vi "GetTriggerTime.vi"() -> (0 "error out":errorcluster, 3 "TriggerTime [ns]":i64)   [LabVIEW 2014]
uses:
  <vilib>/httpClient/LabVIEWHTTPClient.lvlib
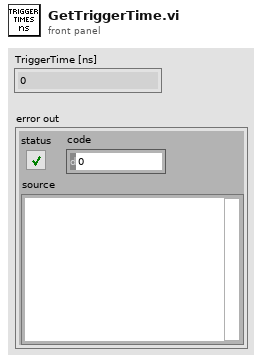
[diagram p1: front panel]
types:
  T1 = typedef "LabVIEWHTTPClient.lvlib/ClientHandle.ctl" = refnum<k1>
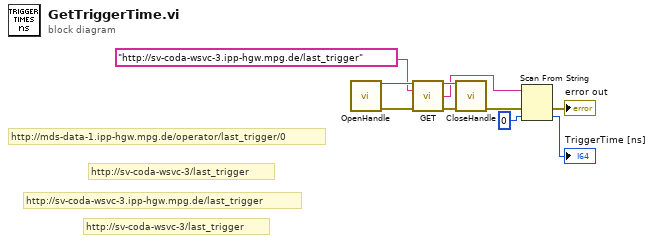
[diagram p0: block diagram]
diagram:
  # "http://sv-coda-wsvc-3/last_trigger"
  # "http://sv-coda-wsvc-3.ipp-hgw.mpg.de/last_trigger"
  # "http://sv-coda-wsvc-3/last_trigger"
  # "http://mds-data-1.ipp-hgw.mpg.de/operator/last_trigger/0"
  n1 = call <vilib>:"OpenHandle.vi"() -> ("client handle out"=w7:T1, "error out"=w2:errorcluster)  [unwired: 14 in]
  n2 = call <vilib>:"GET.vi"("client handle"=w7, "url"="http://sv-coda-wsvc-3.ipp-hgw.mpg.de/last_trigger", "error in (no error)"=w2) -> ("client handle out"=w8:T1, "body"=w4:string, "error out"=w9:errorcluster)  [unwired: 9 in, 1 out]
  n3 = call <vilib>:"CloseHandle.vi"("client handle"=w8, "error in (no error)"=w9) -> ("error out"=w10:errorcluster)  [unwired: 13 in]
  n4 = Scan From String(input string=w4, error in=w10, default 1=i64 0 ("default (0 I32)")) -> (error out=→"error out":errorcluster, output 1=→"TriggerTime [ns]":i64)  [unwired: 2 in, 2 out]
